vi "AlliGator Convert Raw Phasor Plot Data v2 to v3.vi"(8 "Error In":errorcluster, 11 "Raw Phasor Plot Data v2":T1) -> (0 "Error Out":errorcluster, 3 "Raw Phasor Plot Data v3":T4 {"Phasor Metadata"."# Folds" min=1; "Phasor Metadata"."ROI Descriptor"."Contours"."Type" items=["No Selection", "Point", "Line", "Rectangle", "Oval", "Polygon", "Freehand Region", "Annulus", "Unused2", "Unused3", "Broken Line", "Freehand Line", "Rotated Rectangle"]})   [LabVIEW 2021, in "AlliGator Phasor Graph.lvlib"]
doc: "Convert Raw Phasor Plot Data v2 to v3."
uses:
  AlliGator Phasor Graph.lvlib
  AlliGator Raw Phasor Plot Data v3.ctl
  Phasor/Phasor (g, s).ctl
  AlliGator Decay Metadata v3.ctl
  Decay Analysis/Decay Preprocessing/AlliGator Decay Background Subtraction Info.ctl
  Decay Analysis/Decay Preprocessing/AlliGator Baseline Subtraction Method.ctl
  Graphs/XY Graph/XY Graph Plot Shift Parameters.ctl
  Graphs/XY Graph/XY Graph Plot Shift Method.ctl
  Decay Analysis/Decay Preprocessing/AlliGator Decay Extrapolation Parameters.ctl
  AlliGator Raw Phasor Plot Data v2.ctl
  AlliGator Decay Metadata.ctl
  Phasor/Phasor.lvlib
  Decay Analysis/Decay Preprocessing/AlliGator Decay Preprocessing.lvlib
  Graphs/XY Graph/XY Graph Add-Ons.lvlib
panel:
  # "see the AlliGator License on the block diagram (Ctrl+E or Window:Show Block Diagram)"
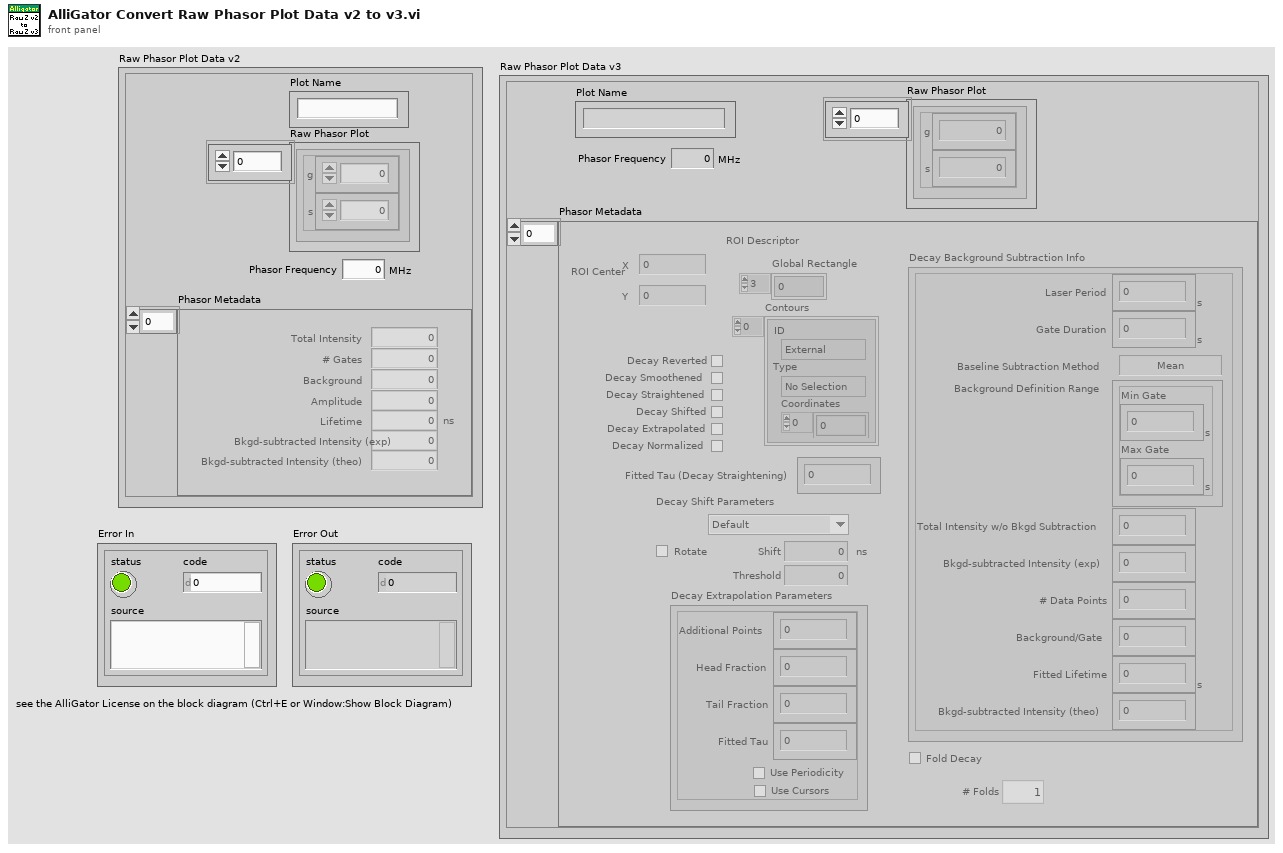
[diagram p1: front panel]
types:
  T1 = typedef "AlliGator Phasor Graph.lvlib/AlliGator Raw Phasor Plot Data v2.ctl" = cluster{"Plot Name":string, "Raw Phasor Plot":T2[], "Phasor Frequency":dbl[unit], "Phasor Metadata":T3[]}
  T2 = typedef "Phasor.lvlib/Phasor (g, s).ctl" = cluster{"g":dbl, "s":dbl}
  T3 = typedef "AlliGator Phasor Graph.lvlib/AlliGator Decay Metadata.ctl" = cluster{"Total Intensity":dbl, "# Gates":i32, "Background":dbl, "Amplitude":dbl, "Lifetime":dbl[unit], "Bkgd-subtracted Intensity (exp)":dbl, "Bkgd-subtracted Intensity (theo)":dbl}
  T4 = typedef "AlliGator Phasor Graph.lvlib/AlliGator Raw Phasor Plot Data v3.ctl" = cluster{"Plot Name":string, "Raw Phasor Plot":T2[], "Phasor Frequency":dbl[unit], "Phasor Metadata":T5[]}
  T5 = typedef "AlliGator Phasor Graph.lvlib/AlliGator Decay Metadata v3.ctl" = cluster{"ROI Descriptor":T6, "ROI Center":cluster{"X":i32, "Y":i32}, "Decay Background Subtraction Info":T7, "Decay Reverted":bool, "Decay Smoothened":bool, "Decay Straightened":bool, "Fitted Tau (Decay Straightening)":dbl, "Decay Shift Parameters":T9, "Decay Shifted":bool, "Decay Extrapolated":bool, "Decay Extrapolation Parameters":T11, "Decay Normalized":bool, "Fold Decay":bool, "# Folds":u32}
  T6 = typedef "ROI Descriptor" = cluster{"Global Rectangle":i32[], "Contours":cluster{"ID":enum32{"External", "Internal"}, "Type":u32, "Coordinates":i32[]}[]}
  T7 = typedef "AlliGator Decay Preprocessing.lvlib/AlliGator Decay Background Subtraction Info.ctl" = cluster{"Laser Period":dbl[unit], "Gate Duration":dbl[unit], "Baseline Subtraction Method":T8, "Background Definition Range":cluster{"Min Gate":dbl[unit], "Max Gate":dbl[unit]}, "Total Intensity w/o Bkgd Subtraction":dbl, "Bkgd-subtracted Intensity (exp)":dbl, "# Data Points":i32, "Background/Gate":dbl, "Fitted Lifetime":dbl[unit], "Bkgd-subtracted Intensity (theo)":dbl}
  T8 = typedef "AlliGator Decay Preprocessing.lvlib/AlliGator Baseline Subtraction Method.ctl" = enum16{"Mean", "Min", "Square Gated Single-Exponential", "File", "Constant"}
  T9 = typedef "XY Graph Add-Ons.lvlib/XY Graph Plot Shift Parameters.ctl" = cluster{"Type":T10, "Shift":dbl[unit], "Threshold":dbl, "Rotate":bool}
  T10 = typedef "XY Graph Add-Ons.lvlib/XY Graph Plot Shift Method.ctl" = enum16{"Default", "CFD", "Threshold", "Cross-Correlation"}
  T11 = typedef "AlliGator Decay Preprocessing.lvlib/AlliGator Decay Extrapolation Parameters.ctl" = cluster{"Additional Points":u32, "Head Fraction":dbl, "Fitted Tau":dbl, "Use Periodicity":bool, "Use Cursors":bool, "Tail Fraction":dbl}
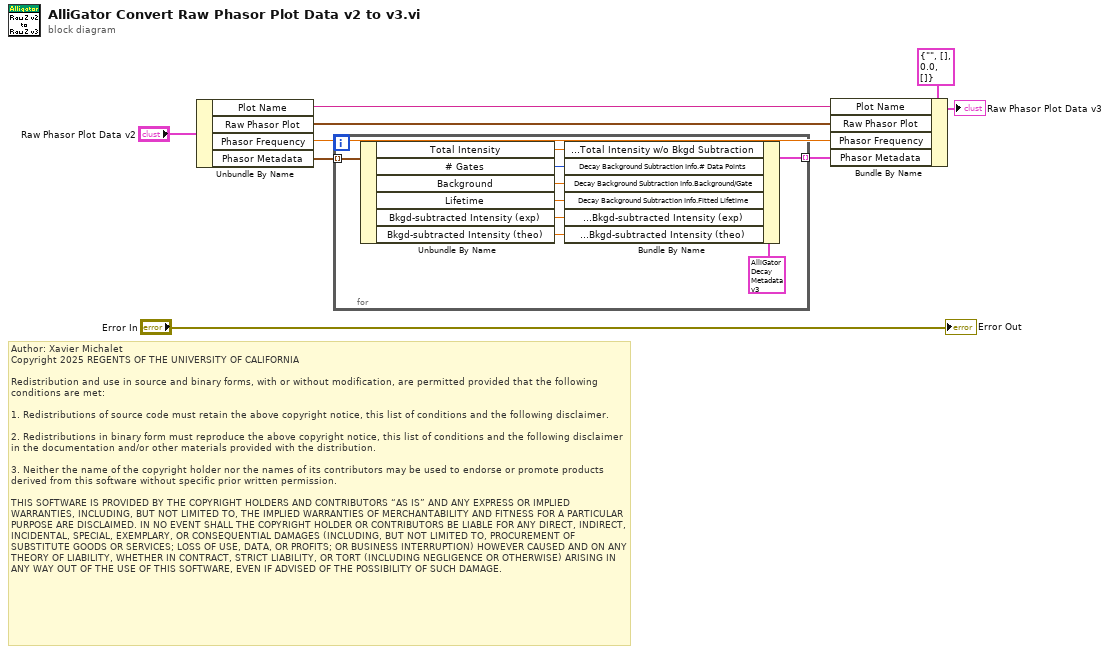
[diagram p0: block diagram]
diagram:
  # "Author: Xavier Michalet\nCopyright 2025 REGENTS OF THE UNIVERSITY OF CALIFORNIA\n\nRedistribution and use in source and binary forms, with or without modification, are permitted provided that the following conditions are met:\n\n1. Redistributions of source code must retain the above copyright notice, this list of conditions and the following disclaimer.\n\n2. Redistributions in binary form must reproduce the above copyright notice, this list of conditions and the following disclaimer in the documentation and/or other materials provided with the distribution.\n\n3. Neither the name of the copyright holder nor the names of its contributors may be used to endorse or promote products derived from this software without specific prior written permission.\n\nTHIS SOFTWARE IS PROVIDED BY THE COPYRIGHT HOLDERS AND CONTRIBUTORS “AS IS” AND ANY EXPRESS OR IMPLIED WARRANTIES, INCLUDING, BUT NOT LIMITED TO, THE IMPLIED WARRANTIES OF MERCHANTABILITY AND FITNESS FOR A PARTICULAR PURPOSE ARE DISCLAIMED. IN NO EVENT SHALL THE COPYRIGHT HOLDER OR CONTRIBUTORS BE LIABLE FOR ANY DIRECT, INDIRECT, INCIDENTAL, SPECIAL, EXEMPLARY, OR CONSEQUENTIAL DAMAGES (INCLUDING, BUT NOT LIMITED TO, PROCUREMENT OF SUBSTITUTE GOODS OR SERVICES; LOSS OF USE, DATA, OR PROFITS; OR BUSINESS INTERRUPTION) HOWEVER CAUSED AND ON ANY THEORY OF LIABILITY, WHETHER IN CONTRACT, STRICT LIABILITY, OR TORT (INCLUDING NEGLIGENCE OR OTHERWISE) ARISING IN ANY WAY OUT OF THE USE OF THIS SOFTWARE, EVEN IF ADVISED OF THE POSSIBILITY OF SUCH DAMAGE."
  n1 = Unbundle By Name("Raw Phasor Plot Data v2") -> ("Plot Name"=w5:string, "Raw Phasor Plot"=w4:T2[], "Phasor Frequency"=w3:dbl[unit], "Phasor Metadata"=w2:T3[])
  n2 = for {
    tunnel: w2 -> [w16] mode=indexing
    tunnel: [w18] -> w1 mode=indexing
    n3 = Unbundle By Name(w16) -> ("Total Intensity"=w15:dbl, "# Gates"=w14:i32, "Background"=w13:dbl, "Lifetime"=w12:dbl[unit], "Bkgd-subtracted Intensity (exp)"=w11:dbl, "Bkgd-subtracted Intensity (theo)"=w10:dbl)
    n4 = Bundle By Name(cluster=T5 {"ROI Descriptor"={"Global Rectangle"=[], "Contours"=[]}, "ROI Center"={"X"=0, "Y"=0}, "Decay Background Subtraction Info"={"Laser Period"=0.0, "Gate Duration"=0.0, "Baseline Subtraction Method"=enum."Mean", "Background Definition Range"={"Min Gate"=0.0, "Max Gate"=0.0}, "Total Intensity w/o Bkgd Subtraction"=0.0, "Bkgd-subtracted Intensity (exp)"=0.0, "# Data Points"=0, "Background/Gate"=0.0, "Fitted Lifetime"=0.0, "Bkgd-subtracted Intensity (theo)"=0.0}, "Decay Reverted"=FALSE, "Decay Smoothened"=FALSE, "Decay Straightened"=FALSE, "Fitted Tau (Decay Straightening)"=0.0, "Decay Shift Parameters"={"Type"=enum."Default", "Shift"=0.0, "Threshold"=0.0, "Rotate"=FALSE}, "Decay Shifted"=FALSE, "Decay Extrapolated"=FALSE, "Decay Extrapolation Parameters"={"Additional Points"=0, "Head Fraction"=0.0, "Fitted Tau"=0.0, "Use Periodicity"=FALSE, "Use Cursors"=FALSE, "Tail Fraction"=0.0}, "Decay Normalized"=FALSE, "Fold Decay"=FALSE, "# Folds"=1} ("Phasor Metadata"), "Decay Background Subtraction Info.Total Intensity w/o Bkgd Subtraction"=w15, "Decay Background Subtraction Info.# Data Points"=w14, "Decay Background Subtraction Info.Background/Gate"=w13, "Decay Background Subtraction Info.Fitted Lifetime"=w12, "Decay Background Subtraction Info.Bkgd-subtracted Intensity (exp)"=w11, "Decay Background Subtraction Info.Bkgd-subtracted Intensity (theo)"=w10) -> (w18:T5)
  }
  n5 = Bundle By Name(cluster=T4 {"Plot Name"="", "Raw Phasor Plot"=[], "Phasor Frequency"=0.0, "Phasor Metadata"=[]} ("Raw Phasor Plot Data"), "Plot Name"=w5, "Raw Phasor Plot"=w4, "Phasor Frequency"=w3, "Phasor Metadata"=w1) -> (→"Raw Phasor Plot Data v3":T4)
  "Error Out" <- "Error In"
